vi "set_com_port.vi"(8 "error in (no error)":errorcluster, 10 "comm port":refnum<visa-resource-name>, 11 "LightSourceMH110124MaiTai in":refnum<class "LightSourceMH110124MaiTai.lvclass">) -> (0 "error out":errorcluster, 3 "LightSourceMH110124MaiTai out":refnum<class "LightSourceMH110124MaiTai.lvclass">)   [LabVIEW 2010, in "LightSourceMH110124MaiTai.lvclass"]
uses:
  LightSourceMH110124MaiTai.lvclass
  LightSourceMH110124MaiTai.lvclass/LightSourceMH110124MaiTai.ctl
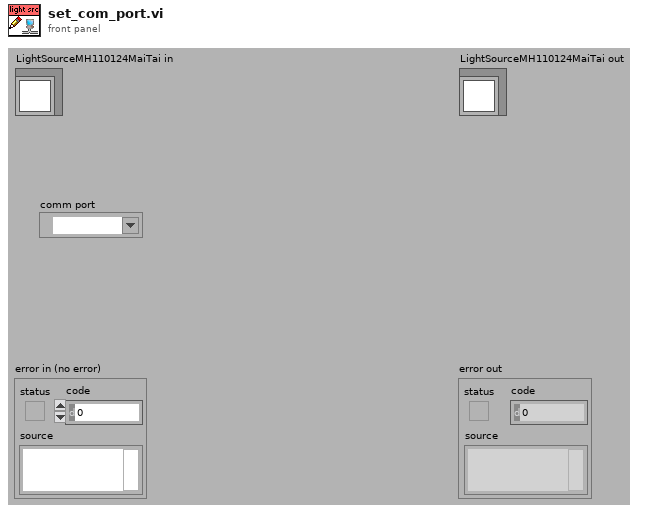
[diagram p1: front panel]
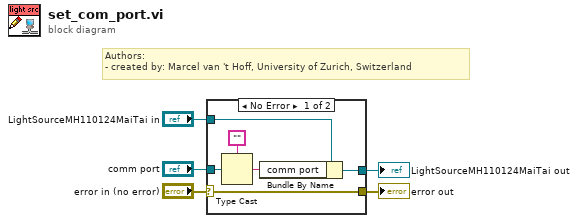
[diagram p0: block diagram]
diagram:
  # "Authors: \n- created by: Marcel van 't Hoff, University of Zurich, Switzerland"
  n1 = case shown="No Error" "error in (no error)" {
    selector: "error in (no error)" -> [w11 w13]
    tunnel: [w11 w13] -> w4
    tunnel: [w6 w12] -> w2
    tunnel: "LightSourceMH110124MaiTai in" -> [w7 w12]
    tunnel: "comm port" -> [w10 _]
    frame No Error {
      n2 = Type Cast(type="", x=w10) -> (*(type *) &x=w8:string)
      n3 = Bundle By Name(cluster=w7, "comm port"=w8) -> (w6:refnum<class "LightSourceMH110124MaiTai.lvclass">)
    }
    frame Error {
    }
  }
  "error out" <- w4
  "LightSourceMH110124MaiTai out" <- w2
